vi "BRig_dataLC_Reward_Trial_l1.vi"() -> (2 "output_Reward_Trial":i32)   [LabVIEW 2014]
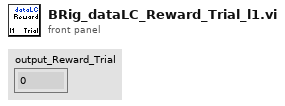
[diagram p1: front panel]
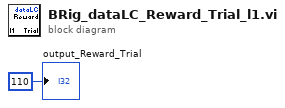
[diagram p0: block diagram]
diagram:
  "output_Reward_Trial" <- 110 ("output_iBlock")
